vi "AnalogDemultiplexer_NI5771_Resonance.vi"() -> ()   [LabVIEW 2012]
uses:
  <vilib>/Platform/TimedLoop/XDataNode/timing_clust.ctl
  <vilib>/Platform/TimedLoop/XDataNode/nitl_modes.ctl
  <vilib>/Platform/TimedLoop/XDataNode/wakeup.ctl
  <vilib>/rvi/FIFO/Fifo_Resource/nirvififoEmulationSetSize.vi
  <vilib>/rvi/DataTransferAndStorage/Container/Common/niFpgaContainerGetUniqueNameForEmu.vi
  <vilib>/rvi/eio/common/nirviEmuTemplateMethod_errors.vi
  <vilib>/rvi/Emulation/niFpgaSctlEmulationRegisterWithScheduler.vi
  <vilib>/rvi/errors/niFpgaSetErrorForExecOnDevCompSimple.vi
  <vilib>/rvi/eio/common/nirviEmuReportErrorAndStop.vi
  <vilib>/rvi/Emulation/niFpgaSctlEmulationFifoFullMgr.vi
  <vilib>/rvi/Emulation/niFpgaSctlEmulationResourceMgr.vi
  <vilib>/rvi/Emulation/niFpgaSctlEmulationScheduler.vi
  <vilib>/rvi/interface/RandomDataEmulation/nirviRandomDataFPGAFIFO.vi
  <vilib>/rvi/interface/RandomDataEmulation/niFpgaRandomDataHandleErrors.vi
  <vilib>/rvi/Emulation/niFpgaSctlEmulationGlobalWrite.vi
  <vilib>/Platform/TimedLoop/XDataNode/XDataNode.xnode
  <vilib>/rvi/DataTransferAndStorage/Container/XNode/niFpgaContainer.xnode
  <vilib>/rvi/FIFO/Fifo_Resource/nirvififoEmulationClear.vi
  <vilib>/eio/EIONode/EIONode.xnode
  <vilib>/rvi/FIFO/Fifo_Resource/nirvififoEmulationWrite.vi
  <vilib>/rvi/FIFO/Fifo_Resource/nirvififoEmulationRead.vi
  <vilib>/rvi/interface/RandomDataEmulation/nirviRandomDataFpgaReadWriteTemplate.vi
  <vilib>/Platform/TimedLoop/XDataNode/XDNodeRunTimeDep.lvlib
panel:
  out "Resonance Trigger":bool
  in  "CutoffU8 Ch2":u8
  in  "CutoffU8 Ch1":u8
  out "ToHostA2FIFO Overflow":bool
  out "ToHostA1FIFO Overflow":bool
  out "Pixel counter A2":u32
  out "Pixel counter A1":u32
  out "InterloopFIFO Overflow":bool
  in  "BaselineU8 Ch2":u8
  in  "BaselineU8 Ch1":u8
  out "InterloopFIFO timeout":bool
  in  "Clear Interloop FIFO":bool
  out "Acquiring":bool
  in  "Wait for trigger":bool
  in  "Acquire":bool
  in  "Requested pixels A2":u32=100000 caption="Requested pixels"
  in  "Acquire continuously":bool=TRUE
  in  "Requested pixels A1":u32=100000 caption="Requested pixels"
  in  "Samples per pixel":u16=10000 caption="Samples per pixel Acq"
  out "IO Module\\AI Over Range":bool
  in  "User Command Commit":bool
  in  "User Command":u8
  out "User Command Idle":bool
  out "User Command Status":u8
  in  "User Data 0":u16
  in  "User Data 1":u8
  out "PLL Locked":bool
  out "User Error":bool
  out "Configured?":bool
  # "5771 IO module configuration"
  # "Analog demultiplexer V2"
  # "Acquisition control"
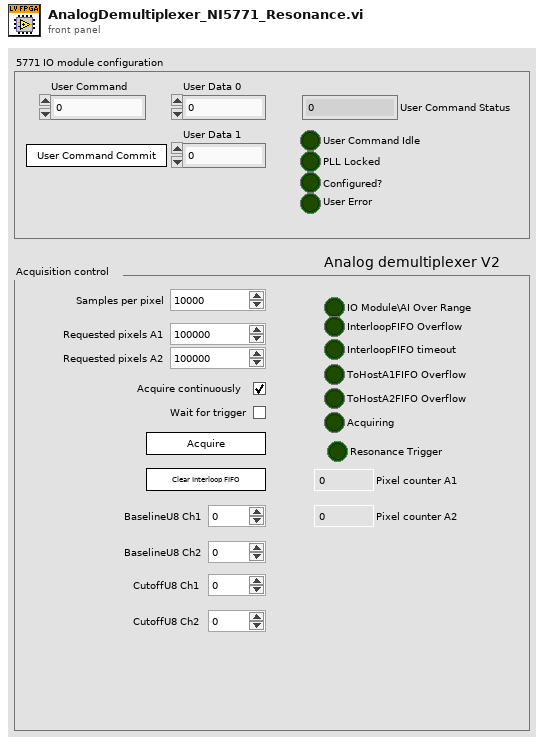
[diagram p1: front panel]
types:
  T1 = typedef "XDNodeRunTimeDep.lvlib/timing_clust.ctl" = cluster{"Expected End [f-1]":u64, "Actual End [f-1]":u64, "Finished Late? [f-1]":bool, "Expected End [i-1]":u64, "Actual End [i-1]":u64, "Finished Late? [i-1]":bool, "Expected Start [i]":u64, "Actual Start [i]":u64, "Expected Start [f]":u64, "Actual Start [f]":u64, "Source Name":string, "Structure Name":string, "Period":i64, "Deadline":i64, "Offset":i64, "Start":i64, "Priority":i32, "Timeout":i32, "Mode":T2, "Wakeup Reason":T3, "Error":errorcluster, "Source Type":string, "Secondary Source Type":string, "Global End Time":u64, "Global Start Time":u64, "Frame Duration":u64, "Iteration Duration":u64, "Assigned CPU":i32, "I/O Scan Engine Mode":u32}
  T2 = typedef "XDNodeRunTimeDep.lvlib/nitl_modes.ctl" = enum32{"No Change", "Process missed periods, maintain original phase", "Discard missed periods, maintain original phase", "Process missed periods, ignore original phase", "Discard missed periods, ignore original phase"}
  T3 = typedef "XDNodeRunTimeDep.lvlib/wakeup.ctl" = enum32{"Normal", "Aborted", "Asynchronous wakeup", "Timing source error", "Timed loop error", "Timeout"}
  T4 = cluster{"IO Module\\AI 1 Data N-7":u8, "IO Module\\AI 1 Data N-6":u8, "IO Module\\AI 1 Data N-5":u8, "IO Module\\AI 1 Data N-4":u8, "IO Module\\AI 1 Data N-3":u8, "IO Module\\AI 1 Data N-2":u8, "IO Module\\AI 1 Data N-1":u8, "IO Module\\AI 1 Data N":u8, "IO Module\\Synchronous Trigger Input":u8}
  T5 = cluster{"IO Module\\AI 0 Data N-7":u8, "IO Module\\AI 0 Data N-6":u8, "IO Module\\AI 0 Data N-5":u8, "IO Module\\AI 0 Data N-4":u8, "IO Module\\AI 0 Data N-3":u8, "IO Module\\AI 0 Data N-2":u8, "IO Module\\AI 0 Data N-1":u8, "IO Module\\AI 0 Data N":u8, "IO Module\\Synchronous Trigger Input":u8}
  T6 = cluster{"Output":u32, "Output":u32, "Output":u32, "Output":u32}
  T7 = cluster{"A1 Ch1":u32, "A1 Ch2":u32, "A2 Ch1":u32, "A2 Ch2":u32}
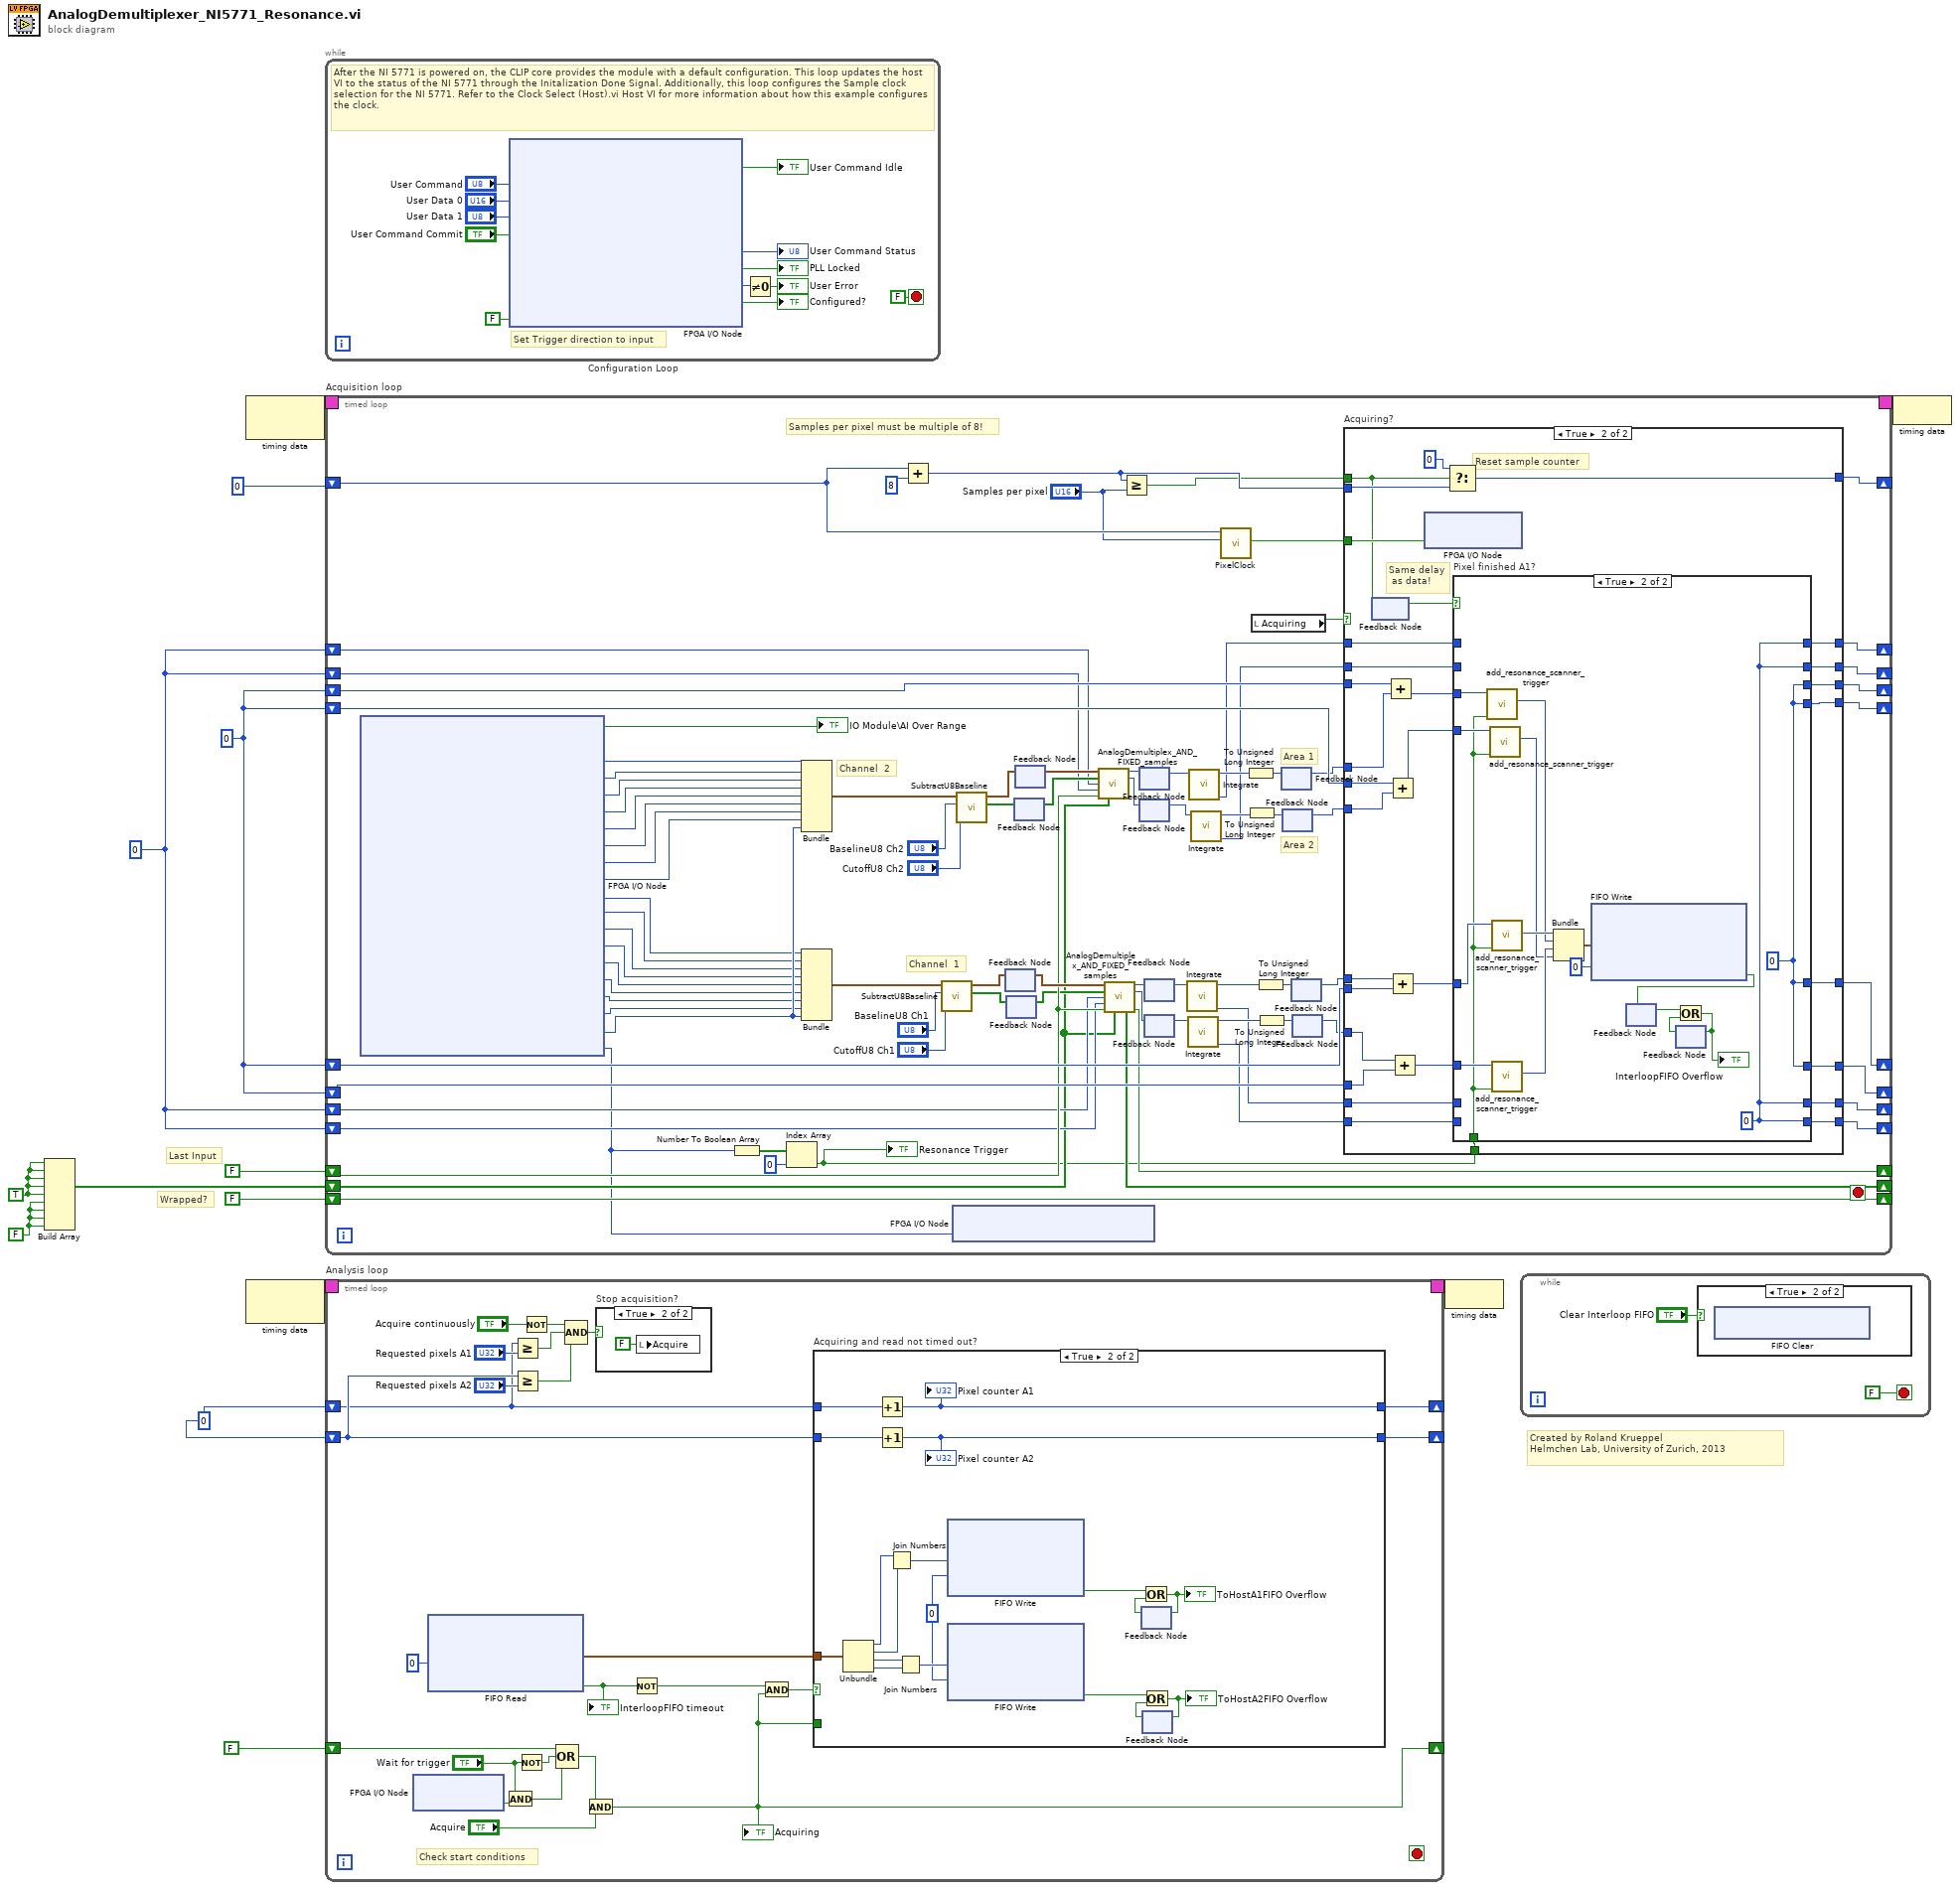
[diagram p0: block diagram]
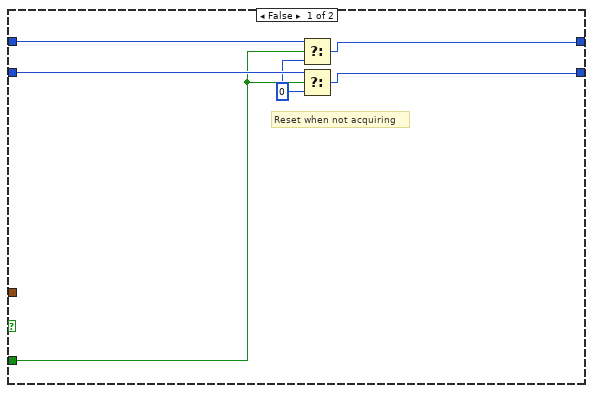
[diagram p3: hidden frame]
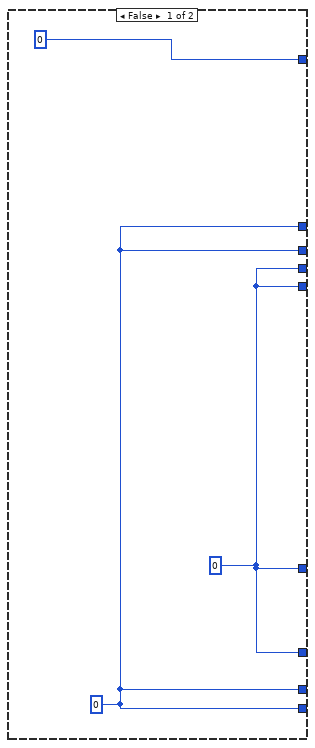
[diagram p5: hidden frame]
diagram:
  w1 = FALSE
  w2 = TRUE
  w4 = u8 0
  w6 = u32 0
  w9 = u32 0 ("Integrator out")
  # "Wrapped?"
  # "Last Input"
  # "Created by Roland Krueppel\nHelmchen Lab, University of Zurich, 2013"
  n1 = Build Array(w2, w2, w2, w2, w2, w1, w1, w1, w1) -> (w3:bool[])
  n2 = node-c288() -> (w14:T1)  [unwired: 1 in]
  n3 = node-c288() -> (w12:T1)  [unwired: 1 in]
  n4 = while "Configuration Loop" {
    stop <- FALSE stop-if-true
    # "Set Trigger direction to input"
    # "After the NI 5771 is powered on, the CLIP core provides the module with a default configuration. This loop updates the host VI to the status of the NI 5771 through the Initalization Done Signal. Additionally, this loop configures the Sample clock selection for the NI 5771. Refer to the Clock Select (Host).vi Host VI for more information about how this example configures the clock."
    n5 = xnode "FPGA I/O Node"("IO Module\\User Command"="User Command", "IO Module\\User Data 0"="User Data 0", "IO Module\\User Data 1"="User Data 1", "IO Module\\User Command Commit"="User Command Commit", "IO Module\\Trigger WE"=FALSE ("IO Module\\Trigger WE")) -> ("IO Module\\User Command Idle"=→"User Command Idle":bool, "IO Module\\User Command Status"=→"User Command Status":u8, "IO Module\\PLL Locked"=→"PLL Locked":bool, "IO Module\\User Error"=w19:u8, "IO Module\\Initialization Done"=→"Configured?":bool)  [unwired: 10 in, 10 out]
    n6 = Not Equal To 0?(x=w19) -> (x != 0?=→"User Error":bool)
  }
  n7 = timed-loop "Acquisition loop" {
    timing: w14 -> [_]
    timing-out: [_] -> w13
    shift-right: [w115] -> _
    shift-left: u16 0 -> [w109]
    shift-right: [w91] -> _
    shift-left: w6 -> [w100]
    shift-right: [w90] -> _
    shift-left: w6 -> [w99]
    shift-right: [w92] -> _
    shift-left: w6 -> [w101]
    shift-right: [w93] -> _
    shift-left: w6 -> [w102]
    shift-right: [w65] -> _
    shift-left: FALSE -> [w75]
    shift-right: [w80] -> _
    shift-left: FALSE -> [w80]
    shift-right: [w72] -> _
    shift-left: w4 -> [w54]
    shift-right: [w71] -> _
    shift-left: w4 -> [w53]
    shift-right: [w74] -> _
    shift-left: w4 -> [w55]
    shift-right: [w73] -> _
    shift-left: w4 -> [w56]
    shift-right: [w52] -> _
    shift-left: w3 -> [w51]
    stop <- _ stop-if-true
    # "Area 2"
    # "Area 1"
    # "Channel  2"
    # "Channel  1"
    # "Samples per pixel must be multiple of 8!"
    n8 = xnode "FPGA I/O Node"() -> ("IO Module\\AI Over Range"=→"IO Module\\AI Over Range":bool, "IO Module\\AI 1 Data N-7"=w46:u8, "IO Module\\AI 1 Data N-6"=w45:u8, "IO Module\\AI 1 Data N-5"=w44:u8, "IO Module\\AI 1 Data N-4"=w43:u8, "IO Module\\AI 1 Data N-3"=w42:u8, "IO Module\\AI 1 Data N-2"=w41:u8, "IO Module\\AI 1 Data N-1"=w40:u8, "IO Module\\AI 1 Data N"=w39:u8, "IO Module\\AI 0 Data N-7"=w37:u8, "IO Module\\AI 0 Data N-6"=w36:u8, "IO Module\\AI 0 Data N-5"=w35:u8, "IO Module\\AI 0 Data N-4"=w34:u8, "IO Module\\AI 0 Data N-3"=w33:u8, "IO Module\\AI 0 Data N-2"=w32:u8, "IO Module\\AI 0 Data N-1"=w31:u8, "IO Module\\AI 0 Data N"=w30:u8, "IO Module\\Synchronous Trigger Input"=w38:u8, "IO Module\\DIO Port 0 Rd Data"=w29:u8)  [unwired: 19 in, 19 out]
    n9 = Number To Boolean Array(number=w29) -> (Boolean array=w28:bool[])
    n10 = Index Array(array=w28, index=0) -> (element=w49:bool)
    "Resonance Trigger" <- w49
    n11 = Bundle("IO Module\\AI 1 Data N-7"=w46, "IO Module\\AI 1 Data N-6"=w45, "IO Module\\AI 1 Data N-5"=w44, "IO Module\\AI 1 Data N-4"=w43, "IO Module\\AI 1 Data N-3"=w42, "IO Module\\AI 1 Data N-2"=w41, "IO Module\\AI 1 Data N-1"=w40, "IO Module\\AI 1 Data N"=w39, "IO Module\\Synchronous Trigger Input"=w38) -> (w47:T4)  [unwired: 1 in]
    n12 = Bundle("IO Module\\AI 0 Data N-7"=w37, "IO Module\\AI 0 Data N-6"=w36, "IO Module\\AI 0 Data N-5"=w35, "IO Module\\AI 0 Data N-4"=w34, "IO Module\\AI 0 Data N-3"=w33, "IO Module\\AI 0 Data N-2"=w32, "IO Module\\AI 0 Data N-1"=w31, "IO Module\\AI 0 Data N"=w30, "IO Module\\Synchronous Trigger Input"=w38) -> (w48:T5)  [unwired: 1 in]
    n13 = Add(x=w109, y=u16 8) -> (x+y=w113:u16)
    n14 = call "SubtractU8Baseline.vi"("Cutoff U8"="CutoffU8 Ch1", "Baseline U8"="BaselineU8 Ch1", "Analog data cluster in"=w48) -> ("Over? Array"=w62:bool[], "Analog data cluster out"=w110:T5)  [unwired: 7 in]
    n15 = xnode "FPGA I/O Node"("IO Module\\DIO Port 1 Wr Data"=w29) -> ()  [unwired: 1 in, 1 out]
    n16 = call "SubtractU8Baseline.vi"("Cutoff U8"="CutoffU8 Ch2", "Baseline U8"="BaselineU8 Ch2", "Analog data cluster in"=w47) -> ("Over? Array"=w64:bool[], "Analog data cluster out"=w111:T5)  [unwired: 7 in]
    n17 = feedback #1() -> (w89:T5)  [unwired: 1 in]
    n18 = feedback-in #1(w110) -> ()
    n19 = feedback #2() -> (w61:bool[])  [unwired: 1 in]
    n20 = feedback-in #2(w62) -> ()
    n21 = feedback #3() -> (w63:bool[])  [unwired: 1 in]
    n22 = feedback-in #3(w64) -> ()
    n23 = feedback-in #4(w111) -> ()
    n24 = feedback #4() -> (w81:T5)  [unwired: 1 in]
    n25 = call "AnalogDemultiplex_AND_FIXED_samples.vi"("Analog data cluster"=w81, "Over? Array"=w63, "Last Sample A1"=w55, "Last Sample A2"=w56, "Last? Input"=w75, "array in"=w51) -> ("Data A1 out"=w85:u64, "Data A2 out"=w83:u64)  [unwired: 6 in, 2 out]
    n26 = call "AnalogDemultiplex_AND_FIXED_samples.vi"("Analog data cluster"=w89, "Over? Array"=w61, "Last Sample A1"=w54, "Last Sample A2"=w53, "Last? Input"=w75, "array in"=w51) -> ("Data A1 out"=w88:u64, "Data A2 out"=w87:u64, "array out"=w52:bool[], "Last? Output"=w65:bool)  [unwired: 6 in]
    n27 = Greater Or Equal?(x=w113, y="Samples per pixel") -> (x >= y?=w112:bool)
    n28 = feedback-in #5(w85) -> ()
    n29 = feedback #5() -> (w84:u64)  [unwired: 1 in]
    n30 = feedback #6() -> (w82:u64)  [unwired: 1 in]
    n31 = feedback-in #6(w83) -> ()
    n32 = feedback #7() -> (w107:u64)  [unwired: 1 in]
    n33 = feedback-in #7(w88) -> ()
    n34 = feedback #8() -> (w86:u64)  [unwired: 1 in]
    n35 = feedback-in #8(w87) -> ()
    n36 = call "Integrate.vi"("New samples in"=w107) -> ("Next Sample"=w67:u8, "Sum out"=w68:u16)  [unwired: 9 in]
    n37 = call "Integrate.vi"("New samples in"=w86) -> ("Next Sample"=w66:u8, "Sum out"=w69:u16)  [unwired: 9 in]
    n38 = call "Integrate.vi"("New samples in"=w84) -> ("Next Sample"=w57:u8, "Sum out"=w60:u16)  [unwired: 9 in]
    n39 = call "Integrate.vi"("New samples in"=w82) -> ("Next Sample"=w58:u8, "Sum out"=w59:u16)  [unwired: 9 in]
    n40 = call "PixelClock.vi"("Samples per pixel"="Samples per pixel", "Sample counter"=w109) -> ("Pixel clock"=w108:bool)  [unwired: 9 in]
    n41 = To Unsigned Long Integer(number=w60) -> (unsigned 32bit integer=w106:u32)
    n42 = To Unsigned Long Integer(number=w59) -> (unsigned 32bit integer=w105:u32)
    n43 = local read "Acquiring"() -> (w94:bool)
    n44 = To Unsigned Long Integer(number=w68) -> (unsigned 32bit integer=w104:u32)
    n45 = To Unsigned Long Integer(number=w69) -> (unsigned 32bit integer=w103:u32)
    n46 = feedback #9() -> (w97:u32)  [unwired: 1 in]
    n47 = feedback-in #9(w106) -> ()
    n48 = feedback #10() -> (w96:u32)  [unwired: 1 in]
    n49 = feedback-in #10(w105) -> ()
    n50 = feedback #11() -> (w98:u32)  [unwired: 1 in]
    n51 = feedback-in #11(w104) -> ()
    n52 = feedback #12() -> (w95:u32)  [unwired: 1 in]
    n53 = feedback-in #12(w103) -> ()
    n54 = case "Acquiring?" shown="True" w94 {
      tunnel: [u16 0 ("t") w149] -> w115
      tunnel: w113 -> [_ w148]
      tunnel: w112 -> [_ w138]
      tunnel: w108 -> [_ w142]
      tunnel: w102 -> [_ w128]
      tunnel: w101 -> [_ w147]
      tunnel: w100 -> [_ w131]
      tunnel: w99 -> [_ w146]
      tunnel: w98 -> [_ w129]
      tunnel: w97 -> [_ w145]
      tunnel: w96 -> [_ w144]
      tunnel: w95 -> [_ w130]
      tunnel: [w118 w136] -> w93
      tunnel: [w118 w135] -> w92
      tunnel: [w118 w134] -> w91
      tunnel: [w118 w133] -> w90
      tunnel: [w116 w127] -> w74
      tunnel: [w116 w126] -> w73
      tunnel: [w116 w125] -> w72
      tunnel: [w116 w124] -> w71
      tunnel: w57 -> [_ w123]
      tunnel: w58 -> [_ w122]
      tunnel: w66 -> [_ w121]
      tunnel: w67 -> [_ w120]
      tunnel: w49 -> [_ w119]
      frame False {
        w116 = u8 0 ("t")
        w118 = u32 0
      }
      frame True {
        # "Same delay\n as data!"
        # "Reset sample counter"
        n55 = feedback #13() -> (w137:bool)  [unwired: 1 in]
        n56 = feedback-in #13(w138) -> ()
        n57 = Add(x=w147, y=w145) -> (x+y=w140:u32)
        n58 = Add(x=w146, y=w144) -> (x+y=w139:u32)
        n59 = Add(x=w129, y=w128) -> (x+y=w141:u32)
        n60 = Add(x=w130, y=w131) -> (x+y=w132:u32)
        n61 = xnode "FPGA I/O Node"("Pixel clock"=w142) -> ()  [unwired: 1 in, 1 out]
        n62 = Select(t=u16 0, s=w138, f=w148) -> (s? t:f=w149:u16)
        n63 = case "Pixel finished A1?" shown="True" w137 {
          tunnel: w141 -> [w157 w165]
          tunnel: w140 -> [w156 w163]
          tunnel: w132 -> [w155 w167]
          tunnel: w139 -> [w154 w161]
          tunnel: [w157 w169] -> w136
          tunnel: [w156 w169] -> w135
          tunnel: [w155 w169] -> w134
          tunnel: [w154 w169] -> w133
          tunnel: [w153 w168] -> w127
          tunnel: [w152 w168] -> w126
          tunnel: [w150 w168] -> w125
          tunnel: [w151 w168] -> w124
          tunnel: w123 -> [w153 _]
          tunnel: w122 -> [w152 _]
          tunnel: w121 -> [w151 _]
          tunnel: w120 -> [w150 _]
          tunnel: w119 -> [_ w159]
          frame False {
          }
          frame True {
            w168 = u8 0
            w169 = u32 0
            n64 = call "add_resonance_scanner_trigger.vi"("Trigger"=w159, "Input"=w163) -> ("Output"=w162:u32)  [unwired: 9 in]
            n65 = call "add_resonance_scanner_trigger.vi"("Trigger"=w159, "Input"=w161) -> ("Output"=w160:u32)  [unwired: 9 in]
            n66 = call "add_resonance_scanner_trigger.vi"("Trigger"=w159, "Input"=w165) -> ("Output"=w164:u32)  [unwired: 9 in]
            n67 = call "add_resonance_scanner_trigger.vi"("Trigger"=w159, "Input"=w167) -> ("Output"=w166:u32)  [unwired: 9 in]
            n68 = Bundle("Output"=w164, "Output"=w162, "Output"=w166, "Output"=w160) -> (w158:T6)  [unwired: 1 in]
            n69 = xnode ("FIFO Write")("Element"=w158, "Timeout"=0) -> ("Timed Out?"=w170:bool)  [unwired: 1 in, 1 out]
            n70 = feedback #14() -> (w171:bool)  [unwired: 1 in]
            n71 = feedback-in #14(w170) -> ()
            n72 = feedback #15() -> (w172:bool)  [unwired: 1 in]
            n73 = Or(x=w171, y=w172) -> (x .or. y?=w173:bool)
            "InterloopFIFO Overflow" <- w173
            n74 = feedback-in #15(w173) -> ()
          }
        }
      }
    }
  }
  n75 = timed-loop "Analysis loop" {
    timing: w12 -> [_]
    timing-out: [_] -> w11
    shift-right: [w177] -> _
    shift-left: FALSE -> [w187]
    shift-right: [w180] -> _
    shift-left: w9 -> [w181]
    shift-right: [w179] -> _
    shift-left: w9 -> [w182]
    stop <- _ stop-if-true
    # "Check start conditions"
    n76 = xnode "FPGA I/O Node"() -> ("TriggerIn"=w192:bool)  [unwired: 1 in, 1 out]
    n77 = xnode ("FIFO Read")("Timeout"=0) -> ("Element"=w178:T7, "Timed Out?"=w184:bool)  [unwired: 1 in, 1 out]
    "InterloopFIFO timeout" <- w184
    n78 = And(x="Wait for trigger", y=w192) -> (x .and. y?=w189:bool)
    n79 = Greater Or Equal?(x=w181, y="Requested pixels A1") -> (x >= y?=w195:bool)
    n80 = Greater Or Equal?(x=w182, y="Requested pixels A2") -> (x >= y?=w194:bool)
    n81 = Not(x="Wait for trigger") -> (.not. x?=w190:bool)
    n82 = Not(x="Acquire continuously") -> (.not. x?=w196:bool)
    n83 = Compound Arithmetic op=OR(w187, w190, w189) -> (w188:bool)
    n84 = Compound Arithmetic op=AND(w196, w195, w194) -> (w186:bool)
    n85 = And(x=w188, y="Acquire") -> (x .and. y?=w177:bool)
    "Acquiring" <- w177
    n86 = case "Stop acquisition?" shown="True" w186 {
      frame False {
      }
      frame True {
        n87 = local write "Acquire"(FALSE ("Acquire")) -> ()
      }
    }
    n88 = Not(x=w184) -> (.not. x?=w183:bool)
    n89 = And(x=w183, y=w177) -> (x .and. y?=w185:bool)
    n90 = case "Acquiring and read not timed out?" shown="True" w185 {
      tunnel: w182 -> [w204 w223]
      tunnel: w181 -> [w206 w224]
      tunnel: [w205 w221] -> w180
      tunnel: [w203 w222] -> w179
      tunnel: w178 -> [_ w220]
      tunnel: w177 -> [w202 _]
      frame False {
        w201 = u32 0 ("f")
        # "Reset when not acquiring"
        n91 = Select(t=w206, s=w202, f=w201) -> (s? t:f=w205:u32)
        n92 = Select(t=w204, s=w202, f=w201) -> (s? t:f=w203:u32)
      }
      frame True {
        w213 = 0 ("Timeout")
        n93 = Unbundle(w220) -> ("A1 Ch1"=w219:u32, "A1 Ch2"=w218:u32, "A2 Ch1"=w216:u32, "A2 Ch2"=w215:u32)
        n94 = Increment(x=w224) -> (x+1=w221:u32)
        "Pixel counter A1" <- w221
        n95 = Increment(x=w223) -> (x+1=w222:u32)
        "Pixel counter A2" <- w222
        n96 = Join Numbers(hi=w219, lo=w218) -> ((hi.lo)=w217:u64)
        n97 = Join Numbers(hi=w216, lo=w215) -> ((hi.lo)=w214:u64)
        n98 = xnode ("FIFO Write")("Element"=w217, "Timeout"=w213) -> ("Timed Out?"=w211:bool)  [unwired: 1 in, 1 out]
        n99 = xnode ("FIFO Write")("Element"=w214, "Timeout"=w213) -> ("Timed Out?"=w207:bool)  [unwired: 1 in, 1 out]
        n100 = feedback #16() -> (w210:bool)  [unwired: 1 in]
        n101 = Or(x=w211, y=w210) -> (x .or. y?=w212:bool)
        "ToHostA1FIFO Overflow" <- w212
        n102 = feedback-in #16(w212) -> ()
        n103 = feedback #17() -> (w208:bool)  [unwired: 1 in]
        n104 = Or(x=w207, y=w208) -> (x .or. y?=w209:bool)
        "ToHostA2FIFO Overflow" <- w209
        n105 = feedback-in #17(w209) -> ()
      }
    }
  }
  n106 = node-c288(w11) -> ()
  n107 = while {
    stop <- FALSE stop-if-true
    n108 = case shown="True" "Clear Interloop FIFO" {
      frame False {
      }
      frame True {
        n109 = xnode ("FIFO Clear")() -> ()  [unwired: 1 in, 1 out]
      }
    }
  }
  n110 = node-c288(w13) -> ()
